vi "setUp.vi"() -> ()   [LabVIEW 2013, in "No Object Control TestCase.lvclass"]
uses:
  No Object Control TestCase.lvclass
panel:
  out "No Object Control TestCase.lvclass 2":refnum<class "No Object Control TestCase.lvclass">
  in  "No Object Control TestCase.lvclass":refnum<class "No Object Control TestCase.lvclass">
  out "error out":errorcluster
  in  "error in (no error)":errorcluster
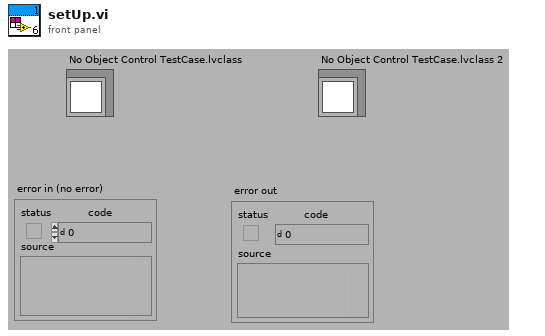
[diagram p1: front panel]
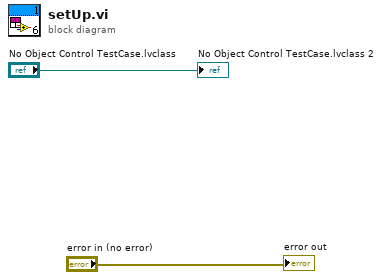
[diagram p0: block diagram]
diagram:
  "error out" <- "error in (no error)"
  "No Object Control TestCase.lvclass 2" <- "No Object Control TestCase.lvclass"
